vi "Com _Defination.vi"(5 "UserNo":string, 6 "TableName":string, 7 "Command":string, 8 "error in (no error)":errorcluster caption="错误输入（无错误）", 9 "FunctionName":string, 10 ".NET:System.Data.DataSet":T1={"CaseSensitive"=FALSE, "Container"=refnum, "DataSetName"="", "DefaultViewManager"=refnum, "DesignMode"=FALSE, "EnforceConstraints"=FALSE, "ExtendedProperties"=refnum, "HasErrors"=FALSE, "IsInitialized"=FALSE, "Locale"=refnum, "Namespace"="", "Prefix"="", "Relations"=refnum, "RemotingFormat"=0, "SchemaSerializationMode"=1, "Site"=refnum, "Tables"=refnum} {"SchemaSerializationMode" items=["IncludeSchema"=1, "ExcludeSchema"=2]; "RemotingFormat" items=["Xml", "Binary"]}, 11 "Traceability 引用句柄":refnum<k24>) -> (0 "error out":errorcluster caption="错误输出", 2 ".NET:System.Data.DataSet":T1={"CaseSensitive"=FALSE, "Container"=refnum, "DataSetName"="", "DefaultViewManager"=refnum, "DesignMode"=FALSE, "EnforceConstraints"=FALSE, "ExtendedProperties"=refnum, "HasErrors"=FALSE, "IsInitialized"=FALSE, "Locale"=refnum, "Namespace"="", "Prefix"="", "Relations"=refnum, "RemotingFormat"=0, "SchemaSerializationMode"=1, "Site"=refnum, "Tables"=refnum} {"SchemaSerializationMode" items=["IncludeSchema"=1, "ExcludeSchema"=2]; "RemotingFormat" items=["Xml", "Binary"]}, 3 "Traceability 引用句柄输出":refnum<k24>)   [LabVIEW 2014, in "Traceability.lvlib"]
uses:
  Traceability.lvlib
  Traceability.dll
  System.Data
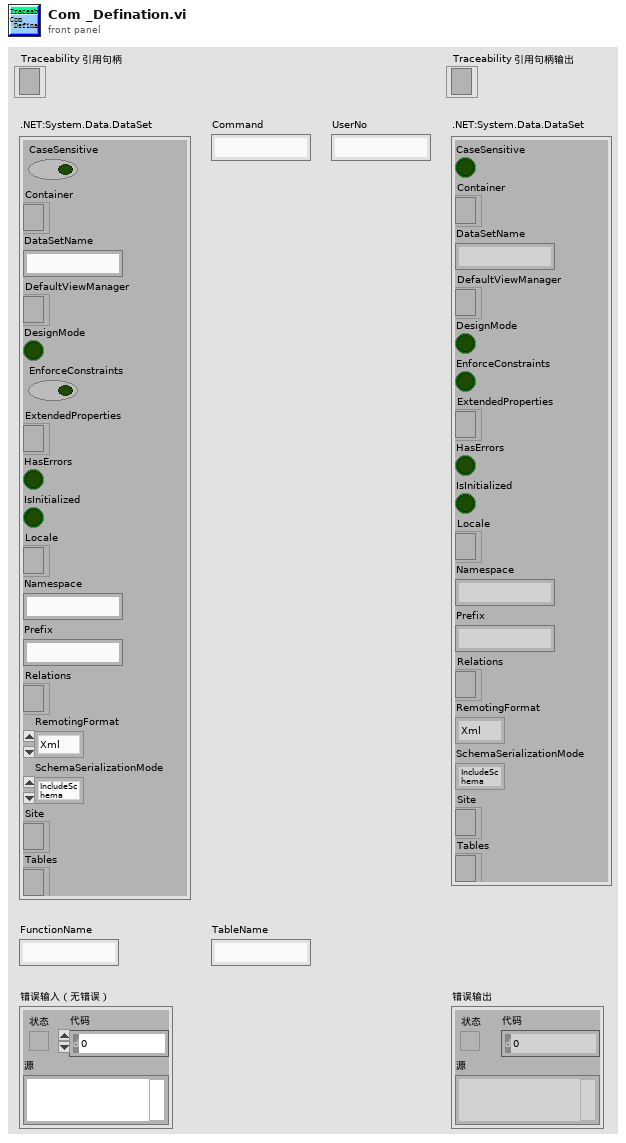
[diagram p1: front panel]
types:
  T1 = cluster{"CaseSensitive":bool, "Container":refnum<k24>, "DataSetName":string, "DefaultViewManager":refnum<k24>, "DesignMode":bool, "EnforceConstraints":bool, "ExtendedProperties":refnum<k24>, "HasErrors":bool, "IsInitialized":bool, "Locale":refnum<k24>, "Namespace":string, "Prefix":string, "Relations":refnum<k24>, "RemotingFormat":i32, "SchemaSerializationMode":i32, "Site":refnum<k24>, "Tables":refnum<k24>}
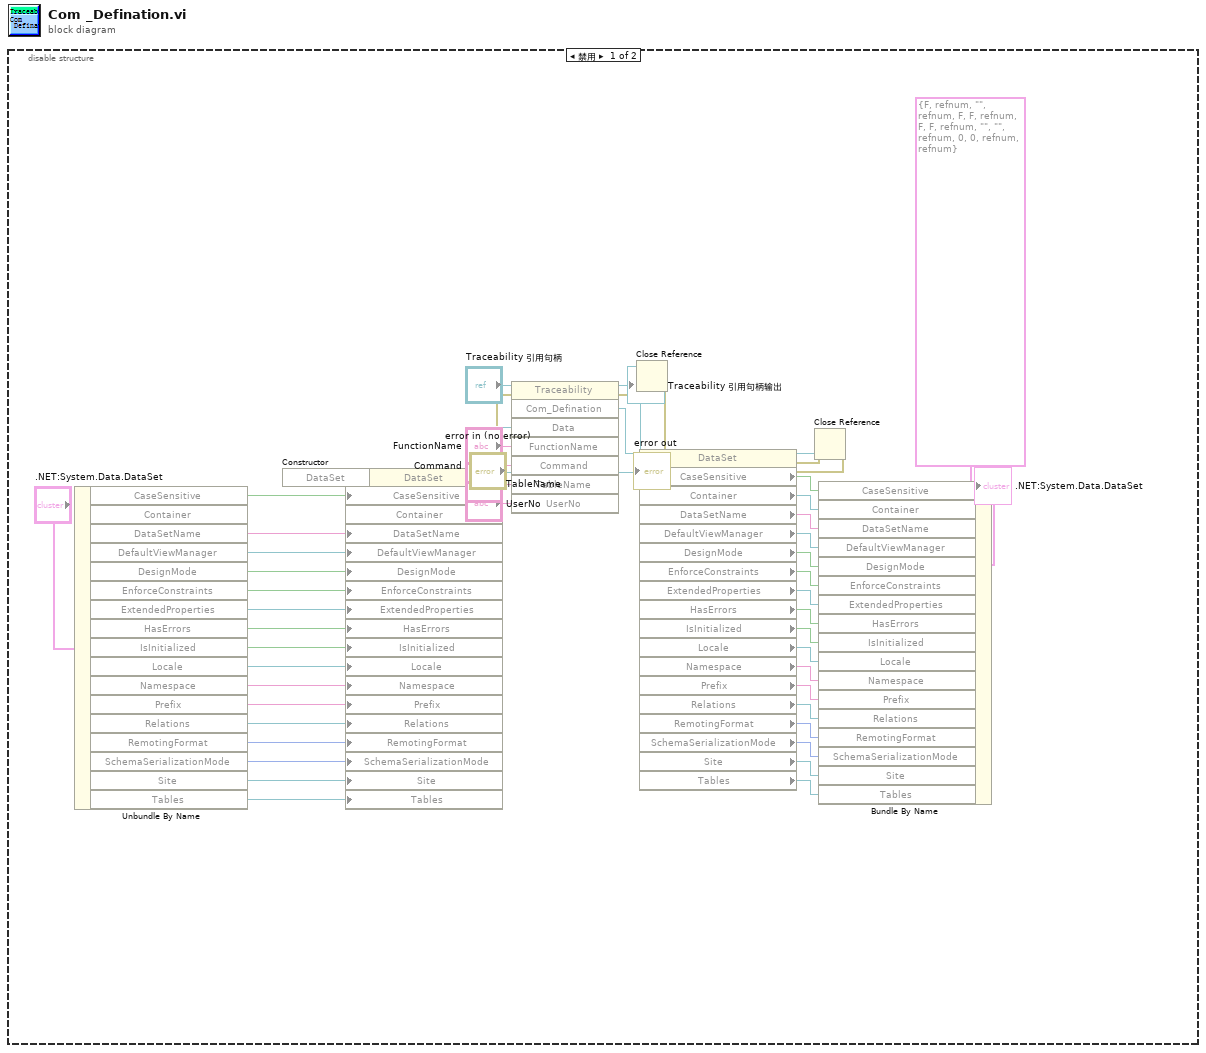
[diagram p0: block diagram]
diagram:
  n1 = disable-structure shown="禁用" {
    frame Disabled {
      n2 = Unbundle By Name(".NET:System.Data.DataSet") -> ("CaseSensitive"=w27:bool, "DataSetName"=w26:string, "DefaultViewManager"=w25:refnum<k24>, "DesignMode"=w24:bool, "EnforceConstraints"=w23:bool, "ExtendedProperties"=w22:refnum<k24>, "HasErrors"=w21:bool, "IsInitialized"=w20:bool, "Locale"=w19:refnum<k24>, "Namespace"=w18:string, "Prefix"=w17:string, "Relations"=w16:refnum<k24>, "RemotingFormat"=w15:i32, "SchemaSerializationMode"=w14:i32, "Site"=w13:refnum<k24>, "Tables"=w12:refnum<k24>)  [unwired: 1 out]
      n3 = constructor class="DataSet"(error in="error in (no error)") -> (reference out=w31:refnum<k24>, error out=w30:errorcluster)  [unwired: 2 in, 1 out]
      n4 = property class="DataSet" props=["CaseSensitive", "Container", "DataSetName", "DefaultViewManager", "DesignMode", "EnforceConstraints", "ExtendedProperties", "HasErrors", "IsInitialized", "Locale", "Namespace", "Prefix", "Relations", "RemotingFormat", "SchemaSerializationMode", "Site", "Tables"](reference=w31, error in=w30, "CaseSensitive"=w27, "DataSetName"=w26, "DefaultViewManager"=w25, "DesignMode"=w24, "EnforceConstraints"=w23, "ExtendedProperties"=w22, "HasErrors"=w21, "IsInitialized"=w20, "Locale"=w19, "Namespace"=w18, "Prefix"=w17, "Relations"=w16, "RemotingFormat"=w15, "SchemaSerializationMode"=w14, "Site"=w13, "Tables"=w12) -> (reference out=w29:refnum<k24>, error out=w6:errorcluster)  [unwired: 1 out]
      n5 = invoke class="Traceability" method="Com_Defination"(reference="Traceability 引用句柄", error in=w6, "Data"=w29, "FunctionName"="FunctionName", "Command"="Command", "TableName"="TableName", "UserNo"="UserNo") -> (reference out=→"Traceability 引用句柄输出":refnum<k24>, error out=w5:errorcluster, "Com_Defination"=w51:refnum<k24>)  [unwired: 1 in, 5 out]
      n6 = Close Reference(reference=w29, error in (no error)=w5) -> (error out=w4:errorcluster)
      n7 = property class="DataSet"(reference=w51, error in=w4) -> (reference out=w3:refnum<k24>, error out=w2:errorcluster, "CaseSensitive"=w48:bool, "Container"=w47:refnum<k24>, "DataSetName"=w46:string, "DefaultViewManager"=w45:refnum<k24>, "DesignMode"=w44:bool, "EnforceConstraints"=w43:bool, "ExtendedProperties"=w42:refnum<k24>, "HasErrors"=w41:bool, "IsInitialized"=w40:bool, "Locale"=w39:refnum<k24>, "Namespace"=w38:string, "Prefix"=w37:string, "Relations"=w36:refnum<k24>, "RemotingFormat"=w35:i32, "SchemaSerializationMode"=w34:i32, "Site"=w33:refnum<k24>, "Tables"=w32:refnum<k24>)
      n8 = Close Reference(reference=w3, error in (no error)=w2) -> (error out=→"error out":errorcluster)
      n9 = Bundle By Name(cluster=T1 {"CaseSensitive"=FALSE, "Container"=refnum, "DataSetName"="", "DefaultViewManager"=refnum, "DesignMode"=FALSE, "EnforceConstraints"=FALSE, "ExtendedProperties"=refnum, "HasErrors"=FALSE, "IsInitialized"=FALSE, "Locale"=refnum, "Namespace"="", "Prefix"="", "Relations"=refnum, "RemotingFormat"=0, "SchemaSerializationMode"=0, "Site"=refnum, "Tables"=refnum} (".NET:System.Data.DataSet"), "CaseSensitive"=w48, "Container"=w47, "DataSetName"=w46, "DefaultViewManager"=w45, "DesignMode"=w44, "EnforceConstraints"=w43, "ExtendedProperties"=w42, "HasErrors"=w41, "IsInitialized"=w40, "Locale"=w39, "Namespace"=w38, "Prefix"=w37, "Relations"=w36, "RemotingFormat"=w35, "SchemaSerializationMode"=w34, "Site"=w33, "Tables"=w32) -> (→".NET:System.Data.DataSet":T1)
    }
    frame Enabled {
    }
  }
